vi "LH-15-07-17.vi"(0 "FPGA VI Reference In":refnum<k20>, 1 "OutputRange":cluster{"output high":dbl, "output low":dbl}[](array[cluster]), 2 "LHSetpoints":dbl[](array[numeric]), 3 "AIsLH":i32[](array[numeric]), 4 "error in":errorcluster, 5 "LH-Gruppe":bool[](array[boolean])=[FALSE, FALSE, FALSE, FALSE, FALSE, FALSE, FALSE, FALSE, FALSE, FALSE, FALSE, FALSE], 6 "PIDs für \"träge\" Heizungen":T1(array[cluster])) -> (7 "error out":errorcluster)   [LabVIEW 2017]
uses:
  GVHeizenLH.vi
  GVAIs.vi
  <vilib>/addons/control/pid/pid.llb/PID (DBL Array).vi
  <vilib>/Utility/error.llb/Error Cluster From Error Code.vi
  <vilib>/rvi/errors/niLvFpgaAdjustHostInterfaceError.vi
  <vilib>/rvi/interface/nirviReadWriteControl/nirviReadWriteControl.xnode
  FPGA Bitfiles/HAGAR-V_FPGATarget_FPGA-Programm-05_gdVwCsZS6sg.lvbitx
  FPGA/FPGA-Programm-05-17.vi
  <vilib>/addons/control/pid/NI_PID_pid.lvlib
  NiFpgaLv.dll
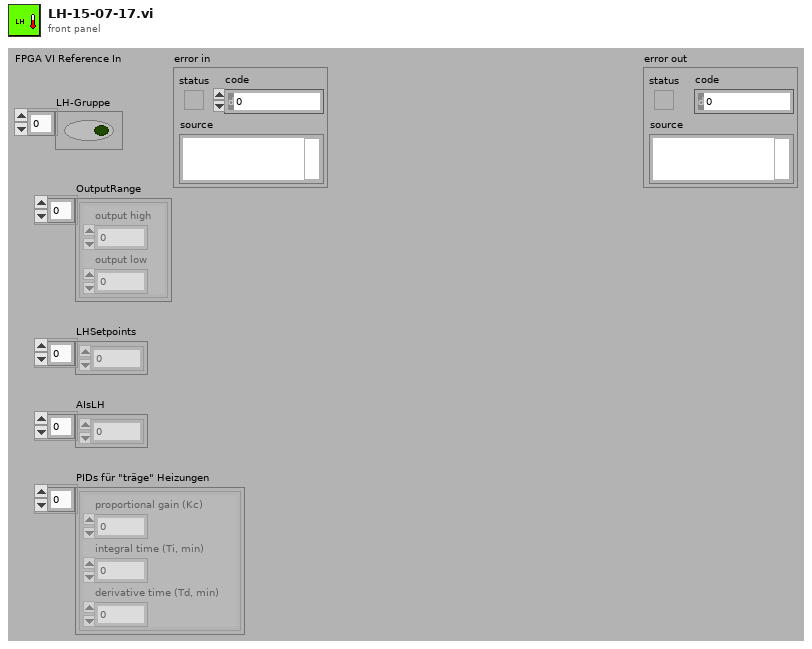
[diagram p1: front panel]
types:
  T1 = cluster{"proportional gain (Kc)":dbl, "integral time (Ti, min)":dbl, "derivative time (Td, min)":dbl}[]
  T2 = cluster{"[0]":bool, "[1]":bool, "[2]":bool, "[3]":bool, "[4]":bool, "[5]":bool, "[6]":bool, "[7]":bool, "[8]":bool, "[9]":bool, "[10]":bool, "[11]":bool, "[12]":bool}
  T3 = cluster{"[0]":u32, "[1]":u32, "[2]":u32, "[3]":u32, "[4]":u32, "[5]":u32, "[6]":u32, "[7]":u32, "[8]":u32, "[9]":u32, "[10]":u32, "[11]":u32, "[12]":u32}
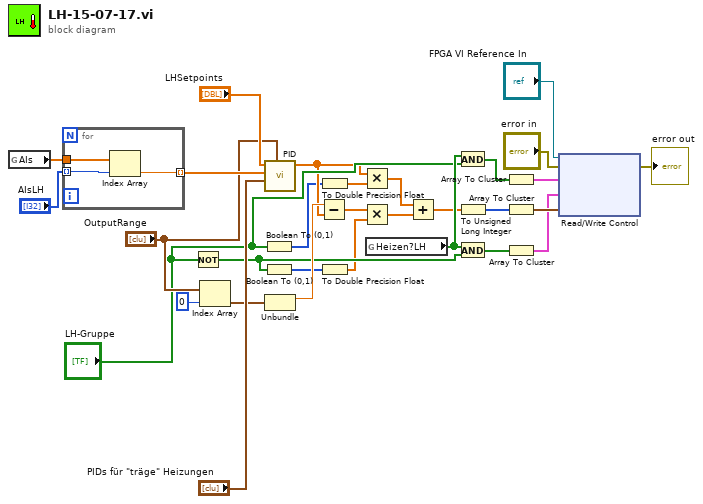
[diagram p0: block diagram]
diagram:
  n1 = global read "GVAIs.vi" "AIs"() -> (w28:dbl[])
  n2 = for {
    tunnel: w28 -> [w33]
    tunnel: "AIsLH" -> [w32] mode=indexing
    tunnel: [w31] -> w24 mode=indexing
    n3 = Index Array(array=w33, index=w32) -> (element=w31:dbl)
  }
  n4 = Not(x="LH-Gruppe") -> (.not. x?=w2:bool[])
  n5 = Index Array(array="OutputRange", index=0) -> (element=w14:cluster{"output high":dbl, "output low":dbl})
  n6 = Boolean To (0,1)(Boolean="LH-Gruppe") -> (0, 1=w10:i16[])
  n7 = Boolean To (0,1)(Boolean=w2) -> (0, 1=w3:i16[])
  n8 = call-poly <vilib>:"PID.vi"("output range"="OutputRange", "PID gains"="PIDs für \"träge\" Heizungen", "process variable"=w24, "setpoint"="LHSetpoints") -> ("output"=w11:dbl[])  [unwired: 6 in, 1 out]
  n9 = Unbundle(w14) -> ("output high"=w12:dbl)  [unwired: 1 out]
  n10 = Subtract(x=w12, y=w11) -> (x-y=w9:dbl[])
  n11 = To Double Precision Float(number=w10) -> (double precision float=w4:dbl[])
  n12 = To Double Precision Float(number=w3) -> (double precision float=w1:dbl[])
  n13 = Multiply(x=w11, y=w4) -> (x*y=w8:dbl[])
  n14 = Multiply(x=w9, y=w1) -> (x*y=w7:dbl[])
  n15 = global read "GVHeizenLH.vi" "Heizen?LH"() -> (w19:bool[])
  n16 = Add(x=w8, y=w7) -> (x+y=w6:dbl[])
  n17 = And(x=w19, y="LH-Gruppe") -> (x .and. y?=w20:bool[])
  n18 = To Unsigned Long Integer(number=w6) -> (unsigned 32bit integer=w5:u32[])
  n19 = And(x=w19, y=w2) -> (x .and. y?=w18:bool[])
  n20 = Array To Cluster(array=w20) -> (cluster=w21:T2)
  n21 = Array To Cluster(array=w5) -> (cluster=w22:T3)
  n22 = Array To Cluster(array=w18) -> (cluster=w17:T2)
  n23 = xnode "Read/Write Control"("FPGA-VI-Referenz (Eingang)"="FPGA VI Reference In", "Fehler (Eingang)"="error in", "LHHeizen1?"=w21, "LHHeizen2?"=w17, "LHPulse(us)"=w22) -> ("Fehler (Ausgang)"=→"error out":errorcluster)  [unwired: 1 out]
